vi "NF87XX.enable driver.vi"(0 "i ref in":refnum<vi>, 1 "System":string="N/A", 2 "Enable Driver":bool, 5 "error in (no error)":errorcluster) -> (14 "i ref out":refnum<vi>, 19 "error out":errorcluster)   [LabVIEW 2014, in "NF87XX.lvlib"]
doc: "Turns on/off all axes channels on the driver. You can still set parameters for disabled drivers but a Move (GO) command will be ignored.\n\nauthor: Stefan Götte\ndata: 09-JAN-2007\n\n\nLicense Agreement for this software:\n\nCopyright (C)\nGesellschaft für Schwerionenforschung, GSI\nPlanckstr. 1\n64291 Darmstadt\nGermany\n\nContact: D.Beck@gsi.de \n\nThis program is free software; you can redistribute it and/or modify it under the terms of the GNU General Public License as published by the Free Software Foundation; either version 2 of the license, or (at your option) any later version.\n\nThis program is distributed in the hope that it will be useful, but WITHOUT ANY WARRANTY; without even the implied warranty of MERCHANTABILITY or FITNESS FOR A PARTICULAR PURPOSE. See the GNU General License for more details (http://www.gnu.org).\n\nGesellschaft für Schwerionenforschung, GSI\nPlanckstr. 1, 64291 Darmstadt, Germany\nFor all questions and ideas contact: M.Richter@gsi.de, H.Brand@gsi.de or D.Beck@gsi.de.\nLast update: 17-JUN-2004"
uses:
  NF87XX.lvlib
  non_GPL/instr.lib/NewFocusPico/Pico Parameters.ctl
  non_GPL/instr.lib/NewFocusPico/NewFocusPico - Driver np.lvlib
panel:
  in  "Pico Parameter type":T1={"Pico Type"=enum."Open-Loop Pico", "Acceleration (steps/sec^2)"="32000", "Velocity ( Hz)"="2000", "Driver"="A1", "Motor"="0", "Channel"="0", "Process Step"="Final Test"}
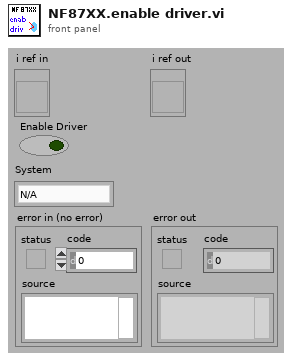
[diagram p1: front panel]
types:
  T1 = typedef "NewFocusPico - Driver np.lvlib/Pico Parameters.ctl" = cluster{"Pico Type":enum16{"Open-Loop Pico", "Close-Loop Pico", "Pico Ultra"}, "Acceleration (steps/sec^2)":string, "Velocity ( Hz)":string, "Driver":string, "Motor":string, "Channel":string, "Process Step":string}
  T2 = enum16{"User....", "DEF", "DIAG", "INI", "LOCK", "UNLOCK", "MAP", "SAV", "VER", "ACC", "CHL", "FOR", "GO", "HAL", "MOF", "MON", "MPV", "POS", "REL", "REV", "STA", "STO", "TYP", "VEL", "ABS", "SER", "NOS", "DRT", "FLI", "RLI", "FIN", "RIN", "AIN", "IN", "JOF", "JON", "OUT", "RES FINE", "RES COARSE", "02 (HEX)", "PWM", "CNT", "TMR", "HOSTNAME", "IPADDR", "IPMODE", "NETMASK", "GATEWAY", "DNSSRVR", "PASSWD", "ECHO", "MACADDR"}
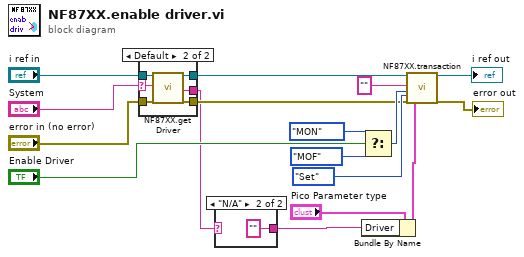
[diagram p0: block diagram]
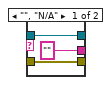
[diagram p2: hidden frame]
diagram:
  n1 = case shown="Default" "System" {
    selector: "System" -> [_ w21]
    tunnel: "i ref in" -> [w20 w26]
    tunnel: "error in (no error)" -> [w19 w25]
    tunnel: [w19 w24] -> w2
    tunnel: [w20 w23] -> w3
    tunnel: ["" ("Driver") w22] -> w1
    frame "", "N/A" {
    }
    frame Default {
      n2 = call "NF87XX.get Driver.vi"("i ref in"=w26, "System"=w21, "error in (no error)"=w25) -> ("i ref out"=w23:refnum<vi>, "Driver"=w22:string, "error out"=w24:errorcluster)  [unwired: 12 in, 2 out]
    }
  }
  n3 = case shown="\"N/A\"" w1 {
    selector: w1 -> [w27 _]
    tunnel: [w27 ""] -> w7
    frame Default {
    }
    frame "N/A" {
    }
  }
  n4 = Bundle By Name(cluster="Pico Parameter type", "Driver"=w7) -> (w11:T1)
  n5 = Select(t=T2."MON" ("MCL Cmd"), s="Enable Driver", f=T2."MOF" ("MCL Cmd")) -> (s? t:f=w8:T2)
  n6 = call "NF87XX.transaction.vi"("i ref in"=w3, "User Cmd/Numeric Argu"="", "MCL Cmd"=w8, "Query/Set"=enum16{"Query", "Set"}."Set", "error in (no error)"=w2, "Pico Parameter"=w11) -> ("i ref out"=→"i ref out":refnum<vi>, "error out"=→"error out":errorcluster)  [unwired: 11 in, 1 out]
